vi "Rigol_Scope_Configure.vi"() -> ()   [LabVIEW 2018]
uses:
  <vilib>/Utility/error.llb/DialogType.ctl
  <instrlib>/RIGOL DS1000 Series/RIGOL DS1000 Series.lvlib
panel:
  out "offsetV":string
  out "offsetT":string
  in  "offsetVoltage":dbl format="%#_6f"
  in  "offsetTime":dbl format="%#_6f"
  out "Command sent":string
  out "chann":string
  out "attn":string
  out "scaleT":string
  out "scaleV":string
  out "bandwidth":string
  out "triggerV":string
  out "filter":string
  in  "F Selector":bool=TRUE
  in  "triggerVoltage":dbl=0.5
  in  "Trigger Type (0: Edge)":u16(ring) items=["Edge", "Pulse", "Video", "Pattern", "Duration"]
  in  "scaleTime":dbl=1.0 format="%#_6f"
  in  "scaleVoltage":dbl=1.0
  in  "BW Selector":bool=TRUE
  in  "Vertical Coupling (0: DC)":u16(ring) items=["DC", "AC", "Ground"]
  in  "Attenuation":i32=500
  in  "Channel (0: Channel 1)":u16(ring) items=["Channel 1", "Channel 2", "Channel 3", "Channel 4"]
  in  "VISA resource name":refnum<visa-resource-name>="USB0::0x1AB1::0x0488::DS1BA202100064::INSTR"
  # "Horizontal"
  # "Probe"
  # "Vertical"
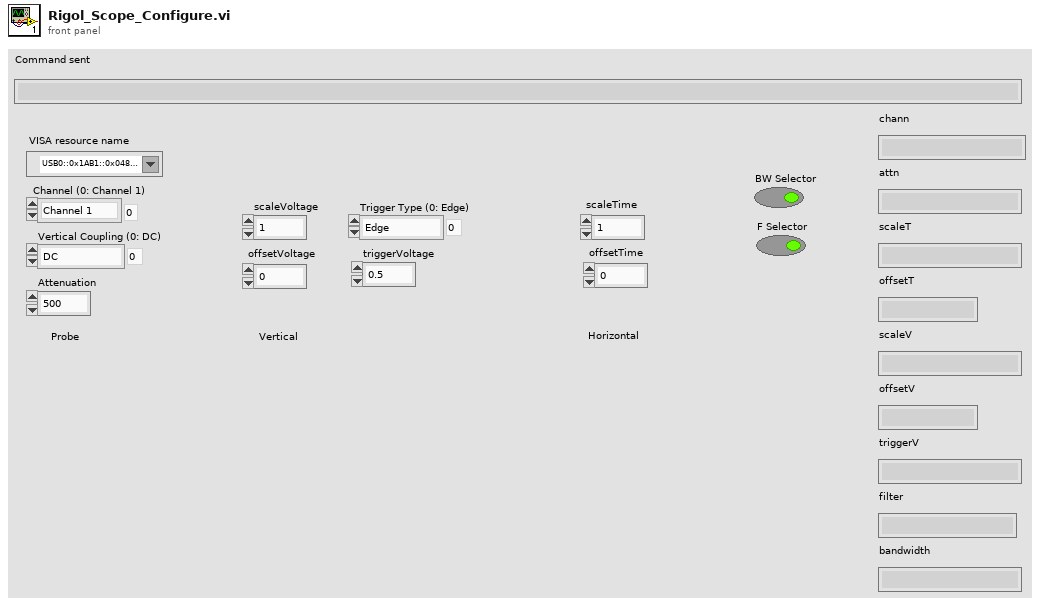
[diagram p1: front panel]
types:
  T1 = typedef "DialogType.ctl" = u16
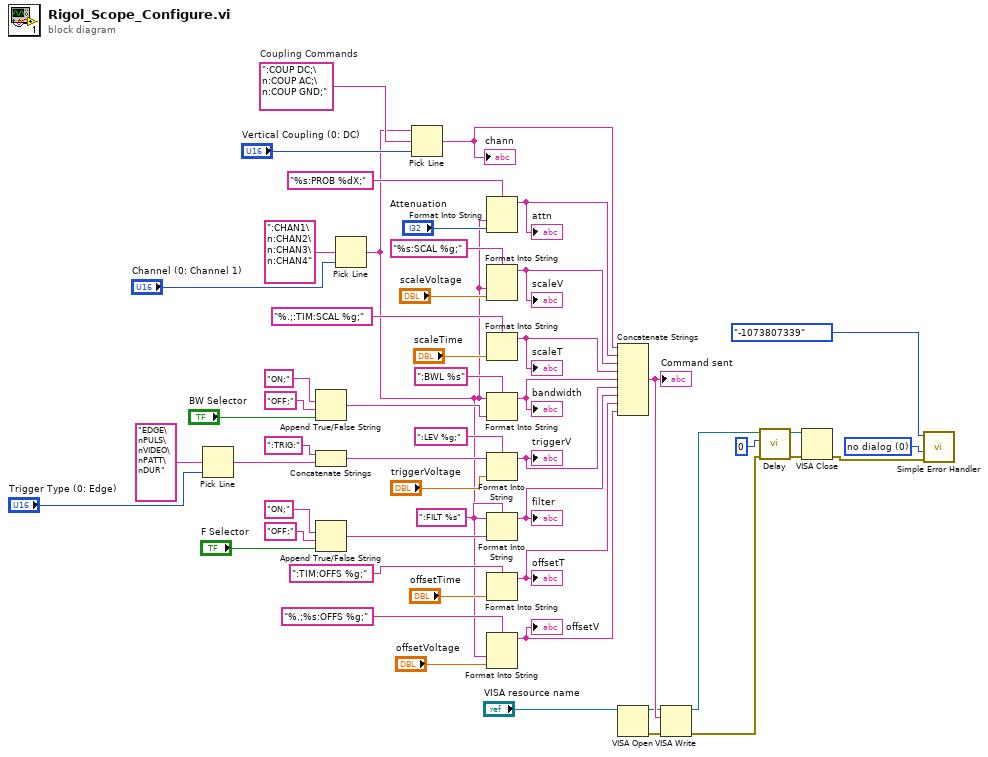
[diagram p0: block diagram]
diagram:
  w11 = T1 0 items=["no dialog", "OK message", "continue or stop message", "OK message + warnings", "continue/stop + warnings"] ("type of dialog (OK msg:1)")
  w45 = ":COUP DC;\n:COUP AC;\n:COUP GND;"  # Coupling Commands
  n1 = Pick Line(multi-line string="EDGE\nPULS\nVIDEO\nPATT\nDUR", line index="Trigger Type (0: Edge)") -> (output string=w38:string)  [unwired: 1 out]
  n2 = Append True/False String(1:"BW Selector", 2:"OFF;" ("false string"), 3:"ON;" ("true string")) -> (0:w42:string)  [unwired: 1 out]
  n3 = Concatenate Strings(":TRIG:" ("string (\"\")"), w38) -> (w32:string)
  n4 = Append True/False String(1:"F Selector", 2:"OFF;" ("false string"), 3:"ON;" ("true string")) -> (0:w28:string)  [unwired: 1 out]
  n5 = Pick Line(multi-line string=":CHAN1\n:CHAN2\n:CHAN3\n:CHAN4" ("多行字符串"), line index="Channel (0: Channel 1)") -> (output string=w1:string)  [unwired: 1 out]
  n6 = Pick Line(string ("")=w1, multi-line string=w45, line index="Vertical Coupling (0: DC)") -> (output string=w25:string)
  "chann" <- w25
  n7 = Format Into String(format string="%s:PROB %dX;", w1, "Attenuation") -> (resulting string=w24:string)  [unwired: 2 in, 1 out]
  "attn" <- w24
  n8 = Format Into String(format string="%s:SCAL %g;", w1, "scaleVoltage") -> (resulting string=w23:string)  [unwired: 2 in, 1 out]
  "scaleV" <- w23
  n9 = Format Into String(format string="%.;:TIM:SCAL %g;", "scaleTime") -> (resulting string=w22:string)  [unwired: 2 in, 1 out]
  "scaleT" <- w22
  n10 = Format Into String(format string=":BWL %s", initial string=w1, w42) -> (resulting string=w21:string)  [unwired: 1 in, 1 out]
  "bandwidth" <- w21
  n11 = Format Into String(format string=":LEV %g;", initial string=w32, "triggerVoltage") -> (resulting string=w20:string)  [unwired: 1 in, 1 out]
  "triggerV" <- w20
  n12 = Format Into String(format string=":FILT %s", initial string=w1, w28) -> (resulting string=w19:string)  [unwired: 1 in, 1 out]
  "filter" <- w19
  n13 = Format Into String(format string=":TIM:OFFS %g;", "offsetTime") -> (resulting string=w7:string)  [unwired: 2 in, 1 out]
  "offsetT" <- w7
  n14 = Format Into String(format string="%.;%s:OFFS %g;", w1, "offsetVoltage") -> (resulting string=w3:string)  [unwired: 2 in, 1 out]
  "offsetV" <- w3
  n15 = Concatenate Strings(w25, w24, w23, w22, w21, w20, w19, w7, w3) -> (w18:string)
  "Command sent" <- w18
  n16 = VISA Open(VISA resource name="VISA resource name") -> (VISA resource name=w16:refnum<visa-resource-name>, error out=w17:errorcluster)  [unwired: 4 in]
  n17 = VISA Write(VISA resource name=w16, write buffer=w18, error in (no error)=w17) -> (VISA resource name out=w15:refnum<visa-resource-name>, error out=w12:errorcluster)  [unwired: 1 out]
  n18 = call <instrlib>:"Delay.vi"("error in (no error)"=w12, "Delay (ms)"=u32 0, "VISA resource name"=w15) -> ("error out"=w13:errorcluster, "VISA resource name out"=w14:refnum<visa-resource-name>)  [unwired: 7 in]
  n19 = VISA Close(VISA resource name=w14, error in (no error)=w13) -> (error out=w9:errorcluster)
  n20 = call <vilib>:"Simple Error Handler.vi"("error code (no error:0)"=enum16{"-1073807339"}."-1073807339", "type of dialog (OK msg:1)"=w11, "error in (no error)"=w9) -> ()  [unwired: 2 in, 5 out]
